vi "PWM.vi"(8 "milliseconds to wait":u32=100, 9 "Period (sec)":dbl=3.0, 10 "Duty Cycle":dbl format="%#_13g", 11 "Starting tic count":u32) -> (2 "Pwm output":dbl, 3 "Elapsed time (sec)":dbl format="%#.3f")   [LabVIEW 2012]
doc: "Use this template to build a standard state machine design pattern. Each state executes code and determines which state to transition to. Contrast this design pattern with the User Interface Event Handler pattern, in which code executes in response to user actions. Contrast this design pattern also with the Queued Message Handler pattern, in which each message handling code can queue zero or more new messages."
panel:
  in  "stop":bool
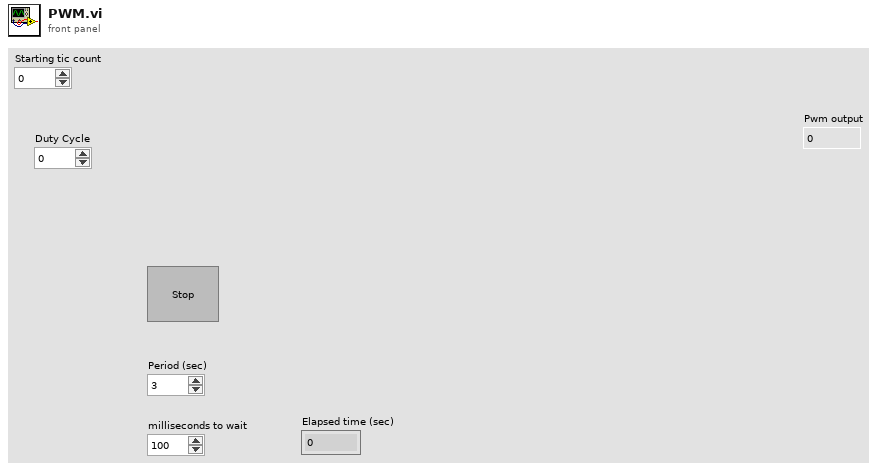
[diagram p1: front panel]
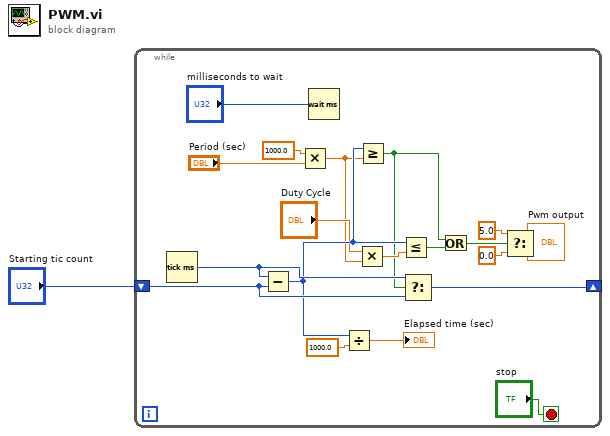
[diagram p0: block diagram]
diagram:
  n1 = while {
    shift-right: [w20] -> _
    shift-left: "Starting tic count" -> [w17]
    stop <- "stop" stop-if-true
    n2 = Tick Count (ms)() -> (millisecond timer value=w12:u32)
    n3 = Subtract(x=w12, y=w17) -> (x-y=w9:u32)
    n4 = Multiply(x=1000.0, y="Period (sec)") -> (x*y=w7:dbl)
    n5 = Wait (ms)(milliseconds to wait="milliseconds to wait") -> ()  [unwired: 1 out]
    n6 = Divide(x=w9, y=1000.0) -> (x/y=→"Elapsed time (sec)":dbl)
    n7 = Multiply(x="Duty Cycle", y=w7) -> (x*y=w6:dbl)
    n8 = Greater Or Equal?(x=w9, y=w7) -> (x >= y?=w3:bool)
    n9 = Less Or Equal?(x=w9, y=w6) -> (x <= y?=w4:bool)
    n10 = Select(t=w12, s=w3, f=w17) -> (s? t:f=w20:u32)
    n11 = Or(x=w3, y=w4) -> (x .or. y?=w5:bool)
    n12 = Select(t=5.0, s=w5, f=0.0) -> (s? t:f=→"Pwm output":dbl)
  }
